vi "Append Lines to Task.vi"(6 "Control":bool, 8 "error in":errorcluster, 10 "lines":tag, 11 "6509 in":refnum<class "6509.lvclass">) -> (0 "error out":errorcluster, 3 "6509 out":refnum<class "6509.lvclass">)   [LabVIEW 2019, in "6509.lvlib" / "6509.lvclass"]
uses:
  Library/6509.lvclass
  Library/6509.lvclass/6509.ctl
  <vilib>/DAQmx/create/channels.llb/DAQmx Create Channel (DO-Digital Output).vi
  <vilib>/DAQmx/create/channels.llb/DAQmx Create Channel (DI-Digital Input).vi
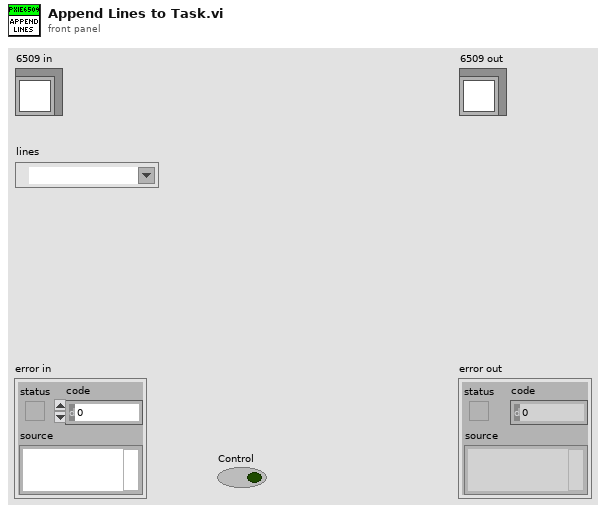
[diagram p1: front panel]
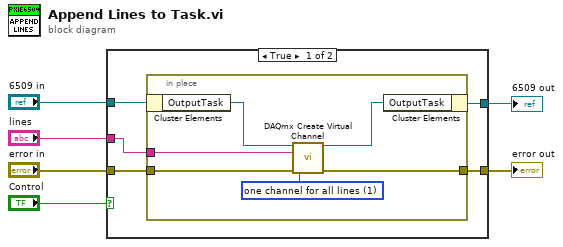
[diagram p0: block diagram]
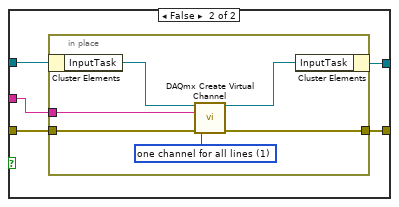
[diagram p2: hidden frame]
diagram:
  n1 = case shown="True" "Control" {
    tunnel: "6509 in" -> [w11 w22]
    tunnel: [w10 w21] -> w5
    tunnel: "lines" -> [w9 w20]
    tunnel: [w8 w19] -> w3
    tunnel: "error in" -> [w7 w18]
    frame True {
      n2 = in-place {
        in-place-border: w9 -> [w15]
        in-place-border: [w13] -> w8
        in-place-border: w7 -> [w12]
        w14 = 1 items=["one channel for each line", "one channel for all lines"] ("line grouping")
        n3 = in-place-cluster #1(w11) -> ("OutputTask"=w17:refnum<k21>)
        n4 = call-poly <vilib>:"DAQmx Create Virtual Channel.vi"("task in"=w17, "lines"=w15, "line grouping"=w14, "error in"=w12) -> ("task out"=w16:refnum<k21>, "error out"=w13:errorcluster)  [unwired: 10 in]
        n5 = in-place-cluster #1("OutputTask"=w16) -> (w10:refnum<class "6509.lvclass">)
      }
    }
    frame False {
      n6 = in-place {
        in-place-border: w20 -> [w26]
        in-place-border: [w24] -> w19
        in-place-border: w18 -> [w23]
        w25 = 1 items=["one channel for each line", "one channel for all lines"] ("line grouping")
        n7 = in-place-cluster #2(w22) -> ("InputTask"=w28:refnum<k21>)
        n8 = call-poly <vilib>:"DAQmx Create Virtual Channel.vi"("task in"=w28, "lines"=w26, "line grouping"=w25, "error in"=w23) -> ("task out"=w27:refnum<k21>, "error out"=w24:errorcluster)  [unwired: 10 in]
        n9 = in-place-cluster #2("InputTask"=w27) -> (w21:refnum<class "6509.lvclass">)
      }
    }
  }
  "error out" <- w3
  "6509 out" <- w5
